vi "motor liste.vi"() -> ()   [LabVIEW 2010]
panel:
  in  "ok":bool
  out "Beschreibung":string="-bitte auswählen-"
  in  "Module":T1(ring)
  in  "Single_Output":T2(ring)
  # "© 2011 Aron Heinecke"
  # "no warranty for this programm"
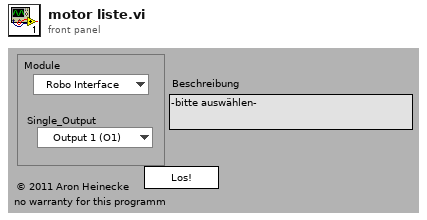
[diagram p1: front panel]
types:
  T1 = enum8{"Robo Interface", "Extension 1", "Extension 2", "Extension 3"}
  T2 = enum8{"Output 1 (O1)", "Output 2 (O2)", "Output 3 (O3)", "Output 4 (O4)", "Output 5 (O5)", "Output 6 (O6)", "Output 7 (O7)", "Output 8 (O8)"}
  T3 = enum8{"Power 1", "Power 2", "Power 3", "Power 4", "Power 5", "Power 6", "Power 7", "Power 8"}
  T4 = enum16{"Device 1", "Device 2", "Device 3", "Device 4", "Device 5", "Device 6", "Device 7", "Device 8"}
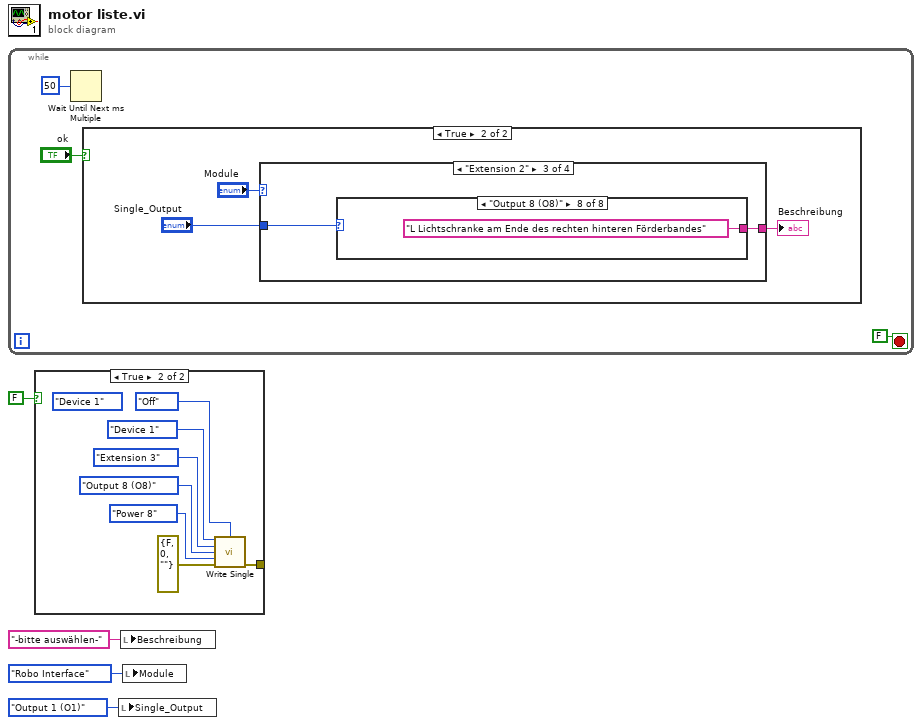
[diagram p0: block diagram]
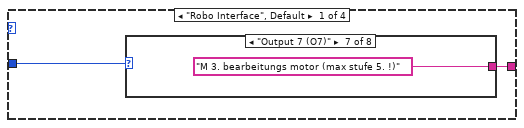
[diagram p4: hidden frame]
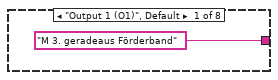
[diagram p5: hidden frame]
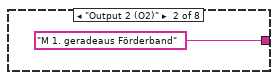
[diagram p6: hidden frame]
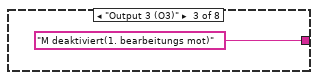
[diagram p7: hidden frame]
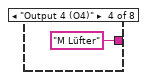
[diagram p8: hidden frame]
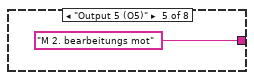
[diagram p9: hidden frame]
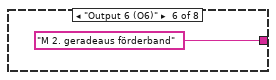
[diagram p10: hidden frame]
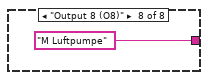
[diagram p11: hidden frame]
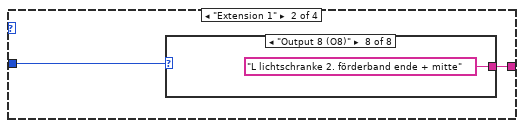
[diagram p12: hidden frame]
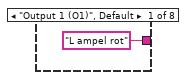
[diagram p13: hidden frame]
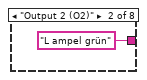
[diagram p14: hidden frame]
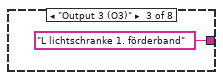
[diagram p15: hidden frame]
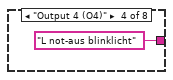
[diagram p16: hidden frame]
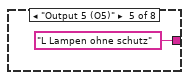
[diagram p17: hidden frame]
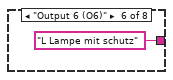
[diagram p18: hidden frame]
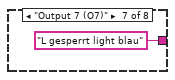
[diagram p19: hidden frame]
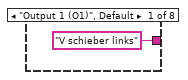
[diagram p20: hidden frame]
diagram:
  n1 = while {
    stop <- FALSE stop-if-true
    n2 = Wait Until Next ms Multiple(millisecond multiple=u32 50 ("Vielfache von ms")) -> ()  [unwired: 1 out]
    n3 = case shown="True" "ok" {
      frame False {
      }
      frame True {
        n4 = case shown="\"Extension 2\"" "Module" {
          tunnel: "Single_Output" -> [w12 w22 w32 w42]
          tunnel: [w11 w21 w31 w41] -> w8
          frame "Robo Interface", Default {
            n5 = case shown="\"Output 7 (O7)\"" w12 {
              tunnel: ["M 3. geradeaus Förderband" "M 1. geradeaus Förderband" "M deaktiviert(1. bearbeitungs mot)" "M Lüfter" "M 2. bearbeitungs mot" "M 2. geradeaus förderband" "M 3. bearbeitungs motor (max stufe 5. !)" "M Luftpumpe"] -> w11
              frame "Output 1 (O1)", Default {
              }
              frame "Output 2 (O2)" {
              }
              frame "Output 3 (O3)" {
              }
              frame "Output 4 (O4)" {
              }
              frame "Output 5 (O5)" {
              }
              frame "Output 6 (O6)" {
              }
              frame "Output 7 (O7)" {
              }
              frame "Output 8 (O8)" {
              }
            }
          }
          frame "Extension 1" {
            n6 = case shown="\"Output 8 (O8)\"" w22 {
              tunnel: ["L ampel rot" "L ampel grün" "L lichtschranke 1. förderband" "L not-aus blinklicht" "L Lampen ohne schutz" "L Lampe mit schutz" "L gesperrt light blau" "L lichtschranke 2. förderband ende + mitte"] -> w21
              frame "Output 1 (O1)", Default {
              }
              frame "Output 2 (O2)" {
              }
              frame "Output 3 (O3)" {
              }
              frame "Output 4 (O4)" {
              }
              frame "Output 5 (O5)" {
              }
              frame "Output 6 (O6)" {
              }
              frame "Output 7 (O7)" {
              }
              frame "Output 8 (O8)" {
              }
            }
          }
          frame "Extension 2" {
            n7 = case shown="\"Output 8 (O8)\"" w32 {
              tunnel: ["V schieber links" "V schieber vorne(raus)" "V schieber rechts" "V sortierung" "L Lichtschranke am Ende des Rechten hinteren Förderbandes" "M Linkes hinteres Förderband" "M Rechtes hinteres Förderband" "L Lichtschranke am Ende des rechten hinteren Förderbandes"] -> w31
              frame "Output 1 (O1)", Default {
              }
              frame "Output 2 (O2)" {
              }
              frame "Output 3 (O3)" {
              }
              frame "Output 4 (O4)" {
              }
              frame "Output 5 (O5)" {
              }
              frame "Output 6 (O6)" {
              }
              frame "Output 7 (O7)" {
              }
              frame "Output 8 (O8)" {
              }
            }
          }
          frame "Extension 3" {
            n8 = case shown="\"Output 5 (O5)\"" w42 {
              tunnel: ["V druckablass" "V" "V" "V" "L lichtschranke 3. geradeaus förderbänder hinten anfang" "L lichtschranke 3. geradeaus förderband ende" "L lichtschranke absperrungs erkennung" "L lichtschranke 1. förderband mitte/ende + 2. förderband anfang"] -> w41
              frame "Output 1 (O1)", Default {
              }
              frame "Output 2 (O2)" {
              }
              frame "Output 3 (O3)" {
              }
              frame "Output 4 (O4)" {
              }
              frame "Output 5 (O5)" {
              }
              frame "Output 6 (O6)" {
              }
              frame "Output 7 (O7)" {
              }
              frame "Output 8 (O8)" {
              }
            }
          }
        }
        "Beschreibung" <- w8
      }
    }
  }
  n9 = case shown="True" FALSE {
    tunnel: [_ w57] -> _
    frame False {
    }
    frame True {
      (unwired) T4."Device 1" ("Device ID Out")
      n10 = call "Write Single.vi"("Device ID"=T4."Device 1", "Output_Action"=enum8{"Off", "On"}."Off", "Module"=T1."Extension 3", "Single_Output"=T2."Output 8 (O8)", "Output_PWM"=T3."Power 8", "error in"=errorcluster {"status"=FALSE, "code"=0, "source"=""}) -> ("error out"=w57:errorcluster)  [unwired: 9 out]
    }
  }
  n11 = local write "Single_Output"(T2."Output 1 (O1)" ("Single_Output")) -> ()
  n12 = local write "Beschreibung"("-bitte auswählen-") -> ()
  n13 = local write "Module"(T1."Robo Interface" ("Module")) -> ()
